vi "NIlib_from_b64.vi"(1 "base64 in":string) -> (0 "string out":string)   [LabVIEW 2023]
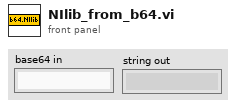
[diagram p1: front panel]
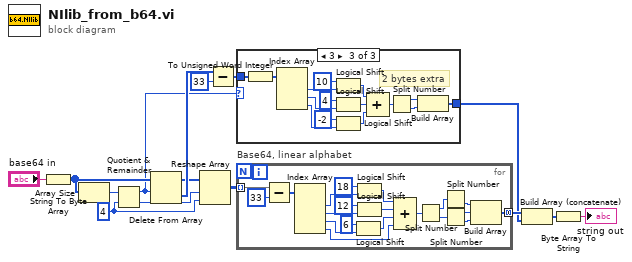
[diagram p0: block diagram]
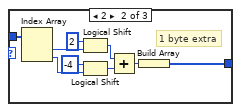
[diagram p3: hidden frame]
diagram:
  w11 = 4 ("y")
  n1 = String To Byte Array(string="base64 in") -> (unsigned byte array=w10:u8[])
  n2 = Array Size(array=w10) -> (size(s)=w13:i32)
  n3 = Quotient & Remainder(x=w13, y=w11) -> (x-y*floor(x/y)=w3:i32, floor(x/y)=w12:i32)
  n4 = Delete From Array(array=w10, length=w3) -> (deleted portion=w9:u8[], array with subset deleted=w7:u8[])  [unwired: 1 in]
  n5 = Reshape Array(w7, w12, w11) -> (w15:u8[][])
  n6 = Subtract(x=w9, y=u8 33 ("x")) -> (x-y=w6:u8[])
  n7 = case shown="3" w3 {
    tunnel: w6 -> [_ w24 w39]
    tunnel: [_ w17 w35] -> w4
    frame 0, Default {
    }
    frame 2 {
      # "1 byte extra"
      n8 = Index Array(array=w24) -> (element #1=w22:u8, element #2=w16:u8)  [unwired: 2 in]
      n9 = Logical Shift(y=i16 2, x=w22) -> (x << y=w20:u8)
      n10 = Logical Shift(y=i16 -4, x=w16) -> (x << y=w19:u8)
      n11 = Add(x=w20, y=w19) -> (x+y=w18:u8)
      n12 = Build Array(w18) -> (w17:u8[])
    }
    frame 3 {
      # "2 bytes extra"
      n13 = To Unsigned Word Integer(number=w39) -> (unsigned 16bit integer=w34:u16[])
      n14 = Index Array(array=w34) -> (element #1=w37:u16, element #2=w33:u16, element #3=w31:u16)  [unwired: 3 in]
      n15 = Logical Shift(y=i16 10, x=w37) -> (x << y=w30:u16)
      n16 = Logical Shift(y=i16 4, x=w33) -> (x << y=w29:u16)
      n17 = Logical Shift(y=i16 -2, x=w31) -> (x << y=w28:u16)
      n18 = Compound Arithmetic op=ADD(w30, w29, w28) -> (w27:u16)
      n19 = Split Number(x=w27) -> (hi(x)=w26:u8, lo(x)=w25:u8)
      n20 = Build Array(w26, w25) -> (w35:u8[])
    }
  }
  n21 = for "Base64, linear alphabet" {
    tunnel: w15 -> [w58] mode=indexing
    tunnel: [w40] -> w5 mode=concatenating
    n22 = Subtract(x=w58, y=u32 33 ("x")) -> (x-y=w57:u32[])
    n23 = Index Array(array=w57) -> (element #1=w56:u32, element #2=w54:u32, element #3=w52:u32, element #4=w47:u32)  [unwired: 4 in]
    n24 = Logical Shift(y=i16 6, x=w52) -> (x << y=w48:u32)
    n25 = Logical Shift(y=i16 18, x=w56) -> (x << y=w50:u32)
    n26 = Logical Shift(y=i16 12, x=w54) -> (x << y=w49:u32)
    n27 = Compound Arithmetic op=ADD(w50, w49, w48, w47) -> (w46:u32)
    n28 = Split Number(x=w46) -> (hi(x)=w45:u16, lo(x)=w44:u16)
    n29 = Split Number(x=w45) -> (lo(x)=w43:u8)  [unwired: 1 out]
    n30 = Split Number(x=w44) -> (hi(x)=w42:u8, lo(x)=w41:u8)
    n31 = Build Array(w43, w42, w41) -> (w40:u8[])
  }
  n32 = Build Array (concatenate)(w5, w4) -> (w14:u8[])
  n33 = Byte Array To String(unsigned byte array=w14) -> (string=→"string out":string)
